vi "PeekElement.vi"(3 "error in (no error)":errorcluster, 5 "Astar Open List in":refnum<class "NI_Robotics_Priority Queue.lvclass">) -> (0 "error out":errorcluster, 1 "Open List Element":T1, 2 "Astar Open List out":refnum<class "NI_Robotics_Priority Queue.lvclass">)   [LabVIEW 2017, in "NI_Robotics_Priority Queue.lvclass"]
uses:
  <vilib>/robotics/Navigation/shared/Priority Queue/NI_Robotics_Priority Queue.lvclass
  <vilib>/robotics/Navigation/shared/Priority Queue/Open List Element.ctl
  <vilib>/robotics/Navigation/shared/MapNode/AbstractMapNode/NI_Robotics_AbstractMapNode.lvclass
  <vilib>/robotics/Navigation/shared/Priority Queue/NI_Robotics_Priority Queue.lvclass/NI_Robotics_Priority Queue.ctl
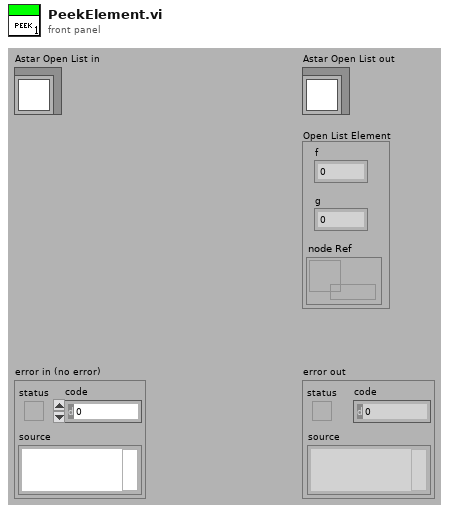
[diagram p1: front panel]
types:
  T1 = typedef "NI_Robotics_Priority Queue.lvclass/Open List Element.ctl" = cluster{"f":dbl, "g":dbl, "node Ref":refnum<data-value>}
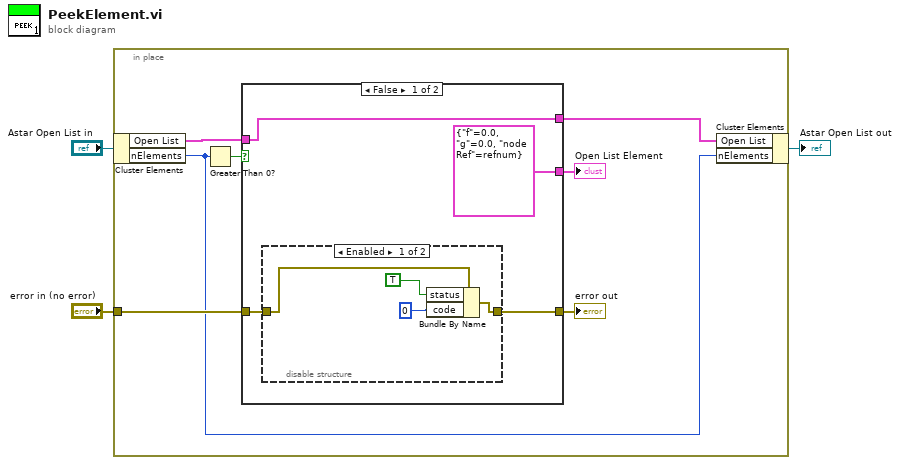
[diagram p0: block diagram]
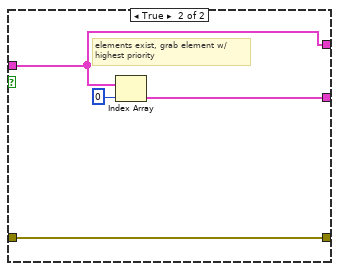
[diagram p3: hidden frame]
diagram:
  n1 = in-place {
    in-place-border: "error in (no error)" -> [w8]
    n2 = in-place-cluster #1("Astar Open List in") -> ("Open List"=w6:T1[], "nElements"=w4:i32)
    n3 = Greater Than 0?(x=w4) -> (x > 0?=w10:bool)
    n4 = case shown="False" w10 {
      tunnel: w6 -> [w11 w20]
      tunnel: [T1 {"f"=0.0, "g"=0.0, "node Ref"=refnum} ("Open List Element") w22] -> w9
      tunnel: w8 -> [w14 w21]
      tunnel: [w13 w21] -> w7
      tunnel: [w11 w20] -> w5
      frame False {
        n5 = disable-structure shown="Enabled" {
          disable-tunnel: w14 -> [w16 w19]
          disable-tunnel: [w15 w19] -> w13
          frame Enabled {
            n6 = Bundle By Name(cluster=w16, "status"=TRUE, "code"=0) -> (w15:errorcluster)
          }
          frame Disabled {
          }
        }
      }
      frame True {
        # "elements exist, grab element w/\nhighest priority"
        n7 = Index Array(array=w20, index=0) -> (element=w22:T1)
      }
    }
    "error out" <- w7
    "Open List Element" <- w9
    n8 = in-place-cluster #1("Open List"=w5, "nElements"=w4) -> (→"Astar Open List out":refnum<class "NI_Robotics_Priority Queue.lvclass">)
  }
